vi "Get_Unique_Labels_from_Folders.vi"(8 "error in (no error)":errorcluster, 11 "Folder Path":path[](array[path])) -> (0 "error out":errorcluster, 3 "Unique_Folders":string[](array[string]))   [LabVIEW 2020]
uses:
  74e48b2f-3ffd-429c-bbef-d590d08817cc.vi
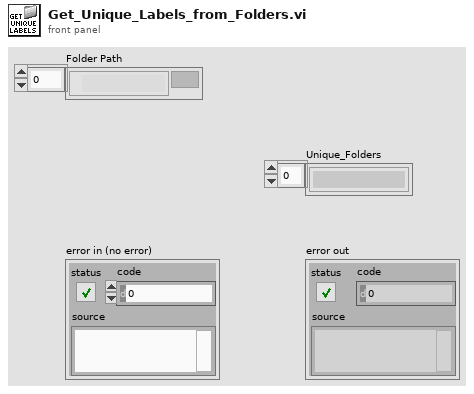
[diagram p1: front panel]
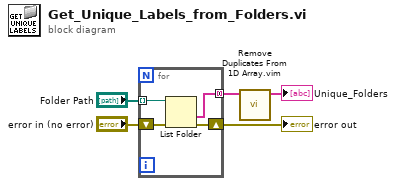
[diagram p0: block diagram]
diagram:
  n1 = for {
    tunnel: [w9] -> w5 mode=concatenating
    tunnel: "Folder Path" -> [w6] mode=indexing
    shift-right: [w8] -> w4
    shift-left: "error in (no error)" -> [w7]
    n2 = List Folder(path=w6, error in=w7) -> (folder names=w9:string[], error out=w8:errorcluster)  [unwired: 2 in, 2 out]
  }
  "error out" <- w4
  n3 = call "Remove Duplicates From 1D Array.vim"("array"=w5) -> ("array with duplicates removed"=→"Unique_Folders":string[])  [unwired: 10 in]
